vi "Status.vi"(8 "error in (no error)":errorcluster, 11 "Response Core in":refnum<class "Interruptible Reply Core.lvclass">) -> (0 "error out":errorcluster, 1 "Time to Timeout (ms)":i32, 2 "Dropped?":bool, 3 "Response Core out":refnum<class "Interruptible Reply Core.lvclass">)   [LabVIEW 2020, in "Publisher.lvlib" / "Interruptible Reply Core.lvclass"]
doc: "Check if the Response Core has been dropped.\n\nThis implementation evaluates the timeout time and checks if the Reply Queue is still valid."
uses:
  Interruptible Reply Core.lvclass
  Interruptible Reply Core.lvclass/Interruptible Reply Core.ctl
  PPL/HDH.Data.Generic.lvlibp/Synchronization/Queue/Queue.lvclass
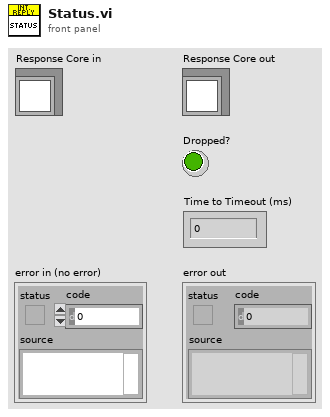
[diagram p1: front panel]
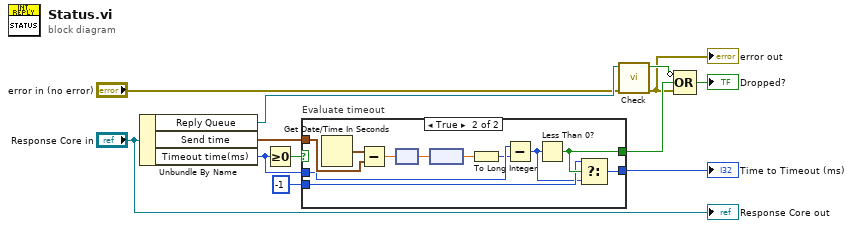
[diagram p0: block diagram]
diagram:
  n1 = Unbundle By Name("Response Core in") -> ("Reply Queue"=w11:refnum<class "Queue.lvclass">, "Send time"=w10:timestamp, "Timeout time(ms)"=w9:i32)
  n2 = Greater Or Equal To 0?(x=w9) -> (x >= 0?=w8:bool)
  n3 = case "Evaluate timeout" shown="True" w8 {
    selector: w8 -> [w14 _]
    tunnel: w10 -> [_ w24]
    tunnel: w9 -> [_ w20]
    tunnel: [w14 w18] -> w5
    tunnel: [w13 w15] -> w1
    tunnel: -1 ("Timeout time(ms)") -> [w13 w17]
    frame False {
    }
    frame True {
      n4 = Get Date/Time In Seconds() -> (seconds since 1Jan1904=w25:timestamp)
      n5 = Subtract(x=w25, y=w24) -> (x-y=w23:dbl)
      n6 = node(w23) -> (w22:dbl[unit])
      n7 = node(w22) -> (w21:dbl)
      n8 = To Long Integer(number=w21) -> (32bit integer=w19:i32)
      n9 = Subtract(x=w20, y=w19) -> (x-y=w16:i32)
      n10 = Less Than 0?(x=w16) -> (x < 0?=w18:bool)
      n11 = Select(t=w17, s=w18, f=w16) -> (s? t:f=w15:i32)
    }
  }
  "Time to Timeout (ms)" <- w1
  n12 = call "Check.vi"("error in (no error)"="error in (no error)", "Queue in"=w11) -> ("error out"=w4:errorcluster, "Queue is valid?"=w7:bool)  [unwired: 8 in]
  "error out" <- w4
  n13 = Compound Arithmetic op=OR(invert w7, w5, w4) -> (→"Dropped?":bool)
  "Response Core out" <- "Response Core in"
